vi "FindSymbol.vi"(8 "error in (no error)":errorcluster, 10 "SymbolName":string, 11 "TCatAdsNet in":refnum<class "AdsNET.lvclass">) -> (0 "error out":errorcluster, 2 "SymbolValue":string, 3 "TCatAdsNet out":refnum<class "AdsNET.lvclass">)   [LabVIEW 2016, in "TCatAdsNet.lvlib" / "AdsNET.lvclass"]
uses:
  AdsNET.lvclass
  AdsNET.lvclass/AdsNET.ctl
  C:/Users/Maurizio/Projects/sentiero-beckoff/DLL/TwinCAT.Ads.dll
  sentiero-beckoff/DLL/TwinCAT.Ads.dll
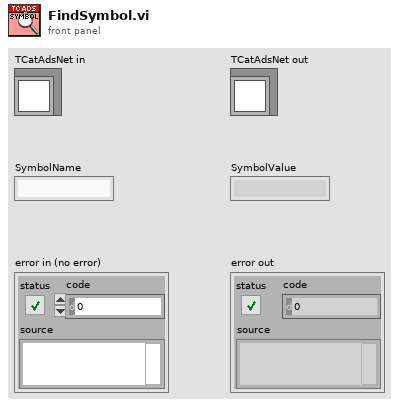
[diagram p1: front panel]
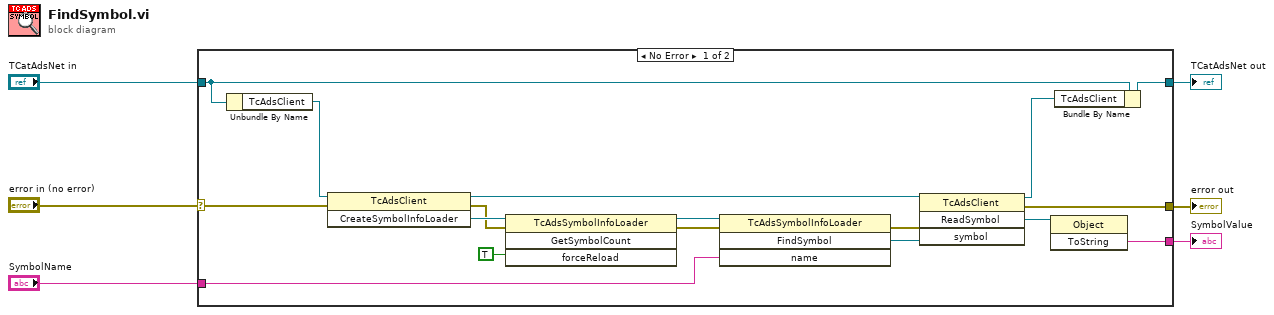
[diagram p0: block diagram]
diagram:
  n1 = case shown="No Error" "error in (no error)" {
    selector: "error in (no error)" -> [w7 w24]
    tunnel: "TCatAdsNet in" -> [w20 w25]
    tunnel: [w19 _] -> w5
    tunnel: [w18 w25] -> w4
    tunnel: [w16 w24] -> w3
    tunnel: "SymbolName" -> [w10 _]
    frame No Error {
      n2 = Unbundle By Name(w20) -> ("TcAdsClient"=w9:refnum<k24>)
      n3 = invoke class="TcAdsClient" method="CreateSymbolInfoLoader"(reference=w9, error in=w7) -> (reference out=w8:refnum<k24>, error out=w13:errorcluster, "CreateSymbolInfoLoader"=w14:refnum<k24>)  [unwired: 1 in]
      n4 = invoke class="TcAdsSymbolInfoLoader" method="GetSymbolCount"(reference=w14, error in=w13, "forceReload"=TRUE) -> (reference out=w12:refnum<k24>, error out=w11:errorcluster)  [unwired: 1 in, 2 out]
      n5 = invoke class="TcAdsSymbolInfoLoader" method="FindSymbol"(reference=w12, error in=w11, "name"=w10) -> (error out=w22:errorcluster, "FindSymbol"=w21:refnum<k24>)  [unwired: 1 in, 2 out]
      n6 = invoke class="TcAdsClient" method="ReadSymbol"(reference=w8, error in=w22, "symbol"=w21) -> (reference out=w17:refnum<k24>, error out=w16:errorcluster, "ReadSymbol"=w23:refnum<k24>)  [unwired: 1 in, 1 out]
      n7 = invoke class="Object" method="ToString"(reference=w23) -> ("ToString"=w19:string)  [unwired: 2 in, 2 out]
      n8 = Bundle By Name(cluster=w20, "TcAdsClient"=w17) -> (w18:refnum<class "AdsNET.lvclass">)
    }
    frame Error {
    }
  }
  "TCatAdsNet out" <- w4
  "error out" <- w3
  "SymbolValue" <- w5
